vi "Pack Step Value.vi"(8 "error in (no error)":errorcluster, 10 "Value":string, 11 "BOOL STEP in":refnum<class "BOOL STEP.lvclass">) -> (0 "error out":errorcluster, 3 "BOOL STEP out":refnum<class "BOOL STEP.lvclass">)   [LabVIEW 2014, in "BOOL STEP.lvlib" / "BOOL STEP.lvclass"]
uses:
  BOOL STEP.lvclass
  BOOL STEP.lvclass/BOOL STEP.ctl
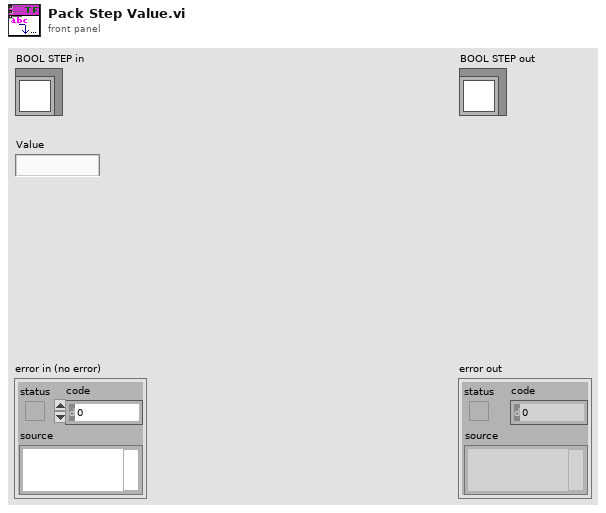
[diagram p1: front panel]
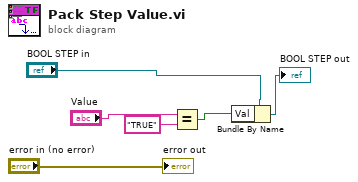
[diagram p0: block diagram]
diagram:
  n1 = Equal?(x="Value", y="TRUE") -> (x = y?=w1:bool)
  n2 = Bundle By Name(cluster="BOOL STEP in", "Val"=w1) -> (→"BOOL STEP out":refnum<class "BOOL STEP.lvclass">)
  "error out" <- "error in (no error)"
